vi "set_ref_clus_ITM10.vi"(6 "cluster_ref":T1, 10 "T":dbl[](array[numeric])=[0.0, 0.0, 0.0, 0.0], 11 "status":bool) -> ()   [LabVIEW 2019]
uses:
  cluster_ref_ITM10.ctl
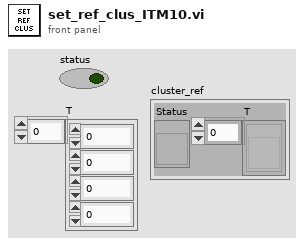
[diagram p1: front panel]
types:
  T1 = typedef "cluster_ref_ITM10.ctl" = cluster{"Status":refnum<vi>, "T":refnum<vi>[]}
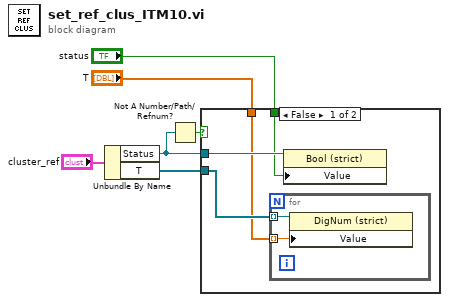
[diagram p0: block diagram]
diagram:
  n1 = Unbundle By Name("cluster_ref") -> ("Status"=w5:refnum<vi>, "T"=w4:refnum<vi>[])
  n2 = Not A Number/Path/Refnum?(number/path/refnum=w5) -> (NaN/Path/Refnum?=w6:bool)
  n3 = case shown="False" w6 {
    tunnel: w5 -> [w10 _]
    tunnel: w4 -> [w8 _]
    tunnel: "status" -> [w9 _]
    tunnel: "T" -> [w7 _]
    frame False {
      n4 = for {
        tunnel: w7 -> [w12] mode=indexing
        tunnel: w8 -> [w11] mode=indexing
        n5 = property class="DigNum (strict)"(reference=w11, "Value"=w12) -> ()  [unwired: 1 in, 2 out]
      }
      n6 = property class="Bool (strict)"(reference=w10, "Value"=w9) -> ()  [unwired: 1 in, 2 out]
    }
    frame True {
    }
  }
